vi "H5Pget_btree_ratios.vi"(6 "error in (no error)":errorcluster, 9 "HDF5 Property Ref":T1) -> (0 "error out":errorcluster, 1 "Right":dbl=0.5 min=0.0 max=1.0, 2 "Left":dbl=0.5 min=0.0 max=1.0, 3 "HDF5 Ref out":T1, 4 "Middle":dbl=0.5 min=0.0 max=1.0)   [LabVIEW 2017]
doc: "Gets B-tree split ratios for a dataset transfer property list."
uses:
  <vilib>/UPVI/lvhdf5/library.llb/HDF5 Ref.ctl
  <vilib>/UPVI/lvhdf5/hdf5.dll
panel:
  # "LVHDF5 Toolkit\nCopyright (c) 2005-2013 by Jason D. Sommerville\nCopyright (c) 2014 by UPVI, LLC.\n\nThis use and distribution of this file is governed by the terms found in \nLICENSE.txt distributed with this toolkit and installed at\n <user.lib>\\_lvhdf5\\LICENSE.txt"
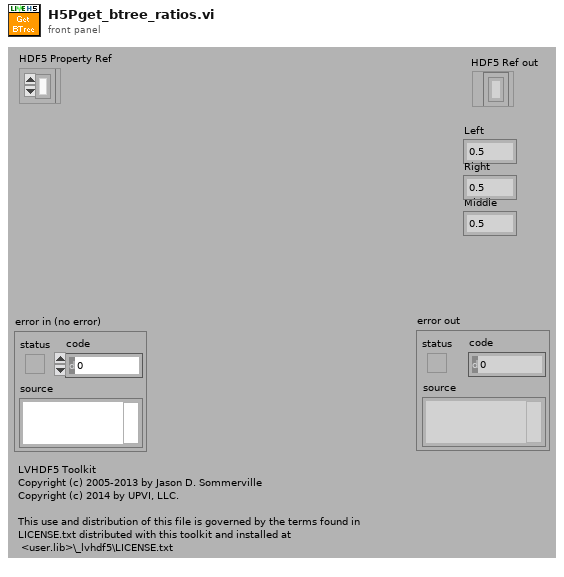
[diagram p1: front panel]
types:
  T1 = typedef "HDF5 Ref.ctl" = refnum<k1>
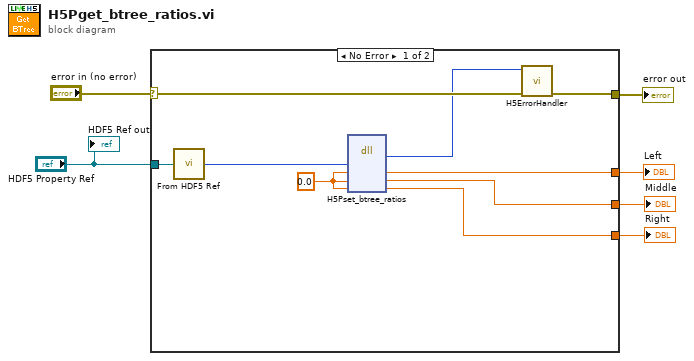
[diagram p0: block diagram]
diagram:
  n1 = case shown="No Error" "error in (no error)" {
    selector: "error in (no error)" -> [w15 w16]
    tunnel: [w14 w16] -> w5
    tunnel: "HDF5 Property Ref" -> [w12 _]
    tunnel: [w9 _] -> w3
    tunnel: [w8 _] -> w2
    tunnel: [w7 _] -> w1
    frame No Error {
      w10 = 0.0 ("left")
      n2 = call <vilib>:"From HDF5 Ref.vi"("HDF5 Ref"=w12) -> ("I32"=w11:i32)
      n3 = dll-call lib="C:/Program Files/National Instruments/LabVIEW 2017/vi.lib/UPVI/lvhdf5/hdf5.dll" fn="H5Pset_btree_ratios" label="H5Pget_btree_ratios"("plist_id"=w11, "left"=w10, "middle"=w10, "right"=w10) -> (w13:i32, "left"=w9:dbl, "middle"=w8:dbl, "right"=w7:dbl)  [unwired: 4 in, 2 out]
      n4 = call <vilib>:"H5ErrorHandler.vi"("error in (no error)"=w15, "herr_t"=w13) -> ("error out"=w14:errorcluster)  [unwired: 3 in, 4 out]
    }
    frame Error {
    }
  }
  "error out" <- w5
  "Left" <- w3
  "Middle" <- w2
  "Right" <- w1
  "HDF5 Ref out" <- "HDF5 Property Ref"
